vi "Get Selected XNET Channels.vi"(8 "error in (no error)":errorcluster, 9 "Node Ptr":u64 format="%.0x", 10 "XNET Cluster":refnum<k21>, 11 "Tree In":refnum<vi>) -> (0 "error out":errorcluster, 3 "Tree Out":refnum<vi>)   [LabVIEW 2019, in "Ghost Bus Addon System Explorer.lvlib"]
uses:
  Ghost Bus Addon System Explorer.lvlib
  <resource>/objmgr/xnet.rc
  <vilib>/NI VeriStand/Custom Device API/Custom Device API.lvlib
panel:
  # "OUTPUTS"
  # "INPUTS"
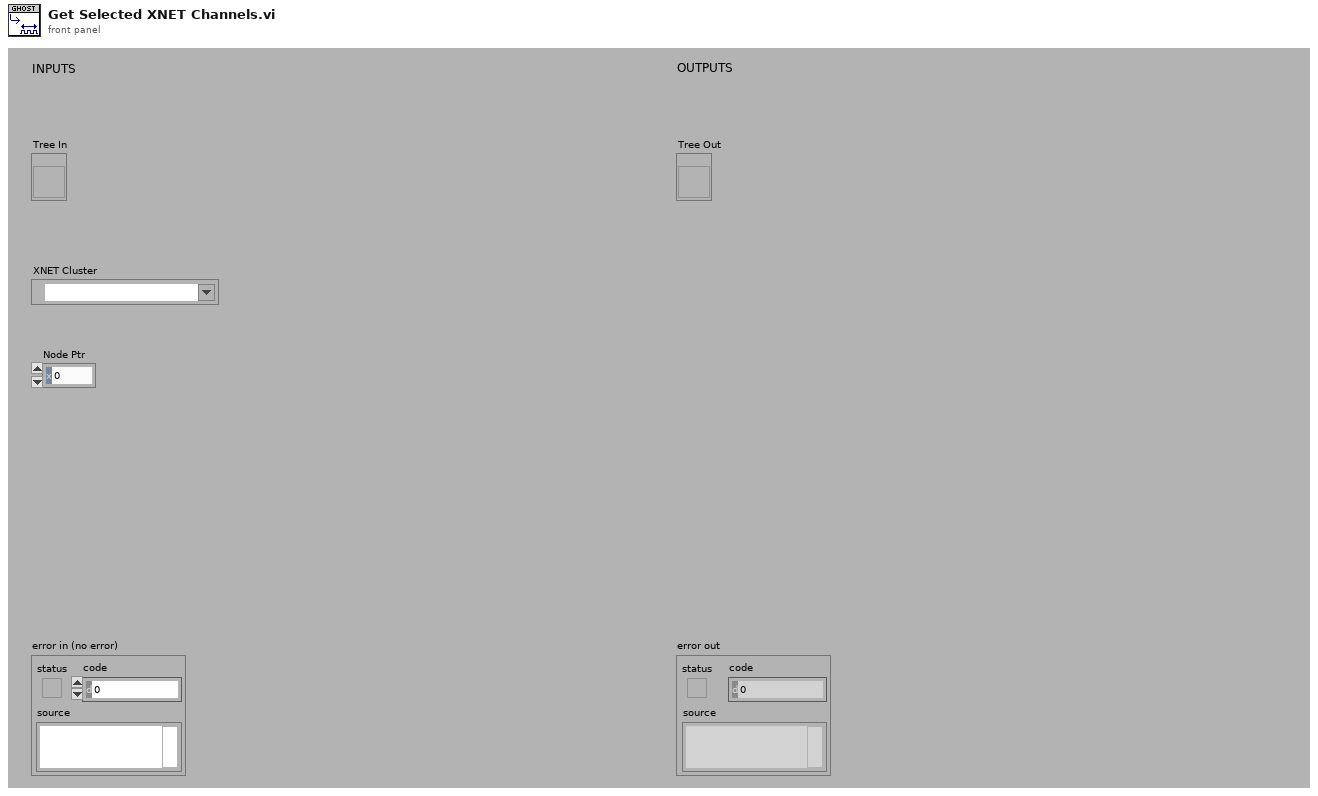
[diagram p1: front panel]
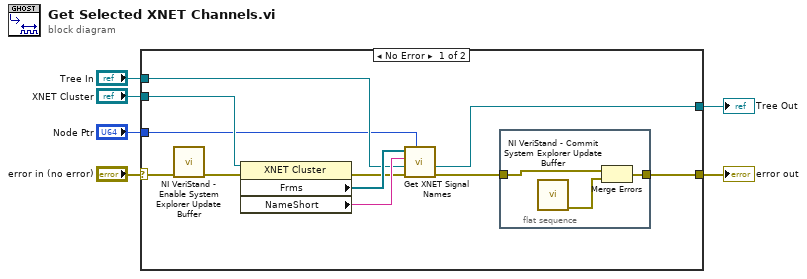
[diagram p0: block diagram]
diagram:
  n1 = case shown="No Error" "error in (no error)" {
    selector: "error in (no error)" -> [w11 w22]
    tunnel: [w9 w22] -> w5
    tunnel: "XNET Cluster" -> [w17 _]
    tunnel: "Tree In" -> [w12 w21]
    tunnel: [w14 w21] -> w2
    tunnel: "Node Ptr" -> [w8 _]
    frame No Error {
      n2 = call <vilib>:"NI VeriStand - Enable System Explorer Update Buffer.vi"("error in (no error)"=w11) -> ("error out"=w7:errorcluster)  [unwired: 10 in]
      n3 = property class="XNET Cluster"(reference=w17, error in=w7) -> (error out=w13:errorcluster, "Frms"=w16:refnum<k21>[], "NameShort"=w15:string)  [unwired: 1 out]
      n4 = call "Get XNET Signal Names.vi"("Parent Ref in"=w8, "error in"=w13, "Tree In"=w12, "Parent"=w15, "Frms"=w16) -> ("error out"=w10:errorcluster, "Tree Out"=w14:refnum<vi>)  [unwired: 5 in]
      n5 = flat-sequence {
        tunnel: w10 -> [w19]
        tunnel: [w18] -> w9
        frame #0 {
          n6 = call <vilib>:"NI VeriStand - Commit System Explorer Update Buffer.vi"() -> ("error out"=w20:errorcluster)  [unwired: 11 in]
          n7 = Merge Errors(w19, w20) -> (w18:errorcluster)
        }
      }
    }
    frame Error {
    }
  }
  "error out" <- w5
  "Tree Out" <- w2
